vi "rcm_pose.vi"(6 "Adjust RCM":bool=TRUE, 9 "Goal positions":sgl[][](array[numeric]), 11 "Nominal positions":sgl[][](array[numeric])) -> (2 "Goal pose (handle basis)":T1 format="%#_4g")   [LabVIEW 2013]
uses:
  <vilib>/Analysis/Matrix/Datatypes/RealMatrix.ctl
  <vilib>/Analysis/baseanly.llb/A x Vector.vi
  utilities/labview/norm_vec_single.vi
  <vilib>/Analysis/baseanly.llb/Real Dot Product.vi
  <vilib>/Analysis/baseanly.llb/Real A x B.vi
  <vilib>/Analysis/NI_AALBase.lvlib
  <vilib>/Analysis/Matrix/NI_Matrix.lvlib
panel:
  out "Adjusted RCM Goal":sgl[](array[numeric])
  out "Calibrated length":sgl
  out "Goal length":sgl
  out "Adjustment unit vector":dbl[](array[numeric]) format="%.2f"
  out "RCM transform":T1 format="%#_3f"
  out "Relative motion (RCM)":T1 format="%#_3f"
  out "Goal in RCM coords":sgl[][](array[numeric])
  # "Debugging:"
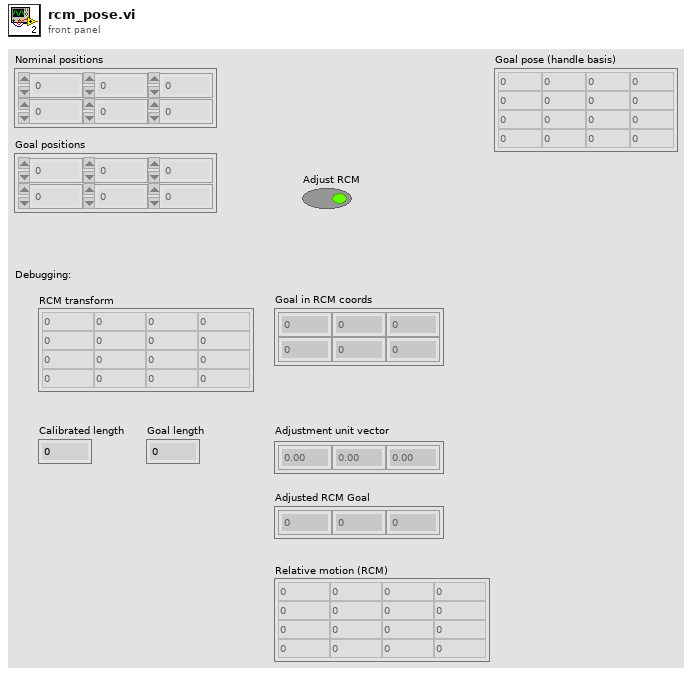
[diagram p1: front panel]
types:
  T1 = typedef "NI_Matrix.lvlib/RealMatrix.ctl" = dbl[][]
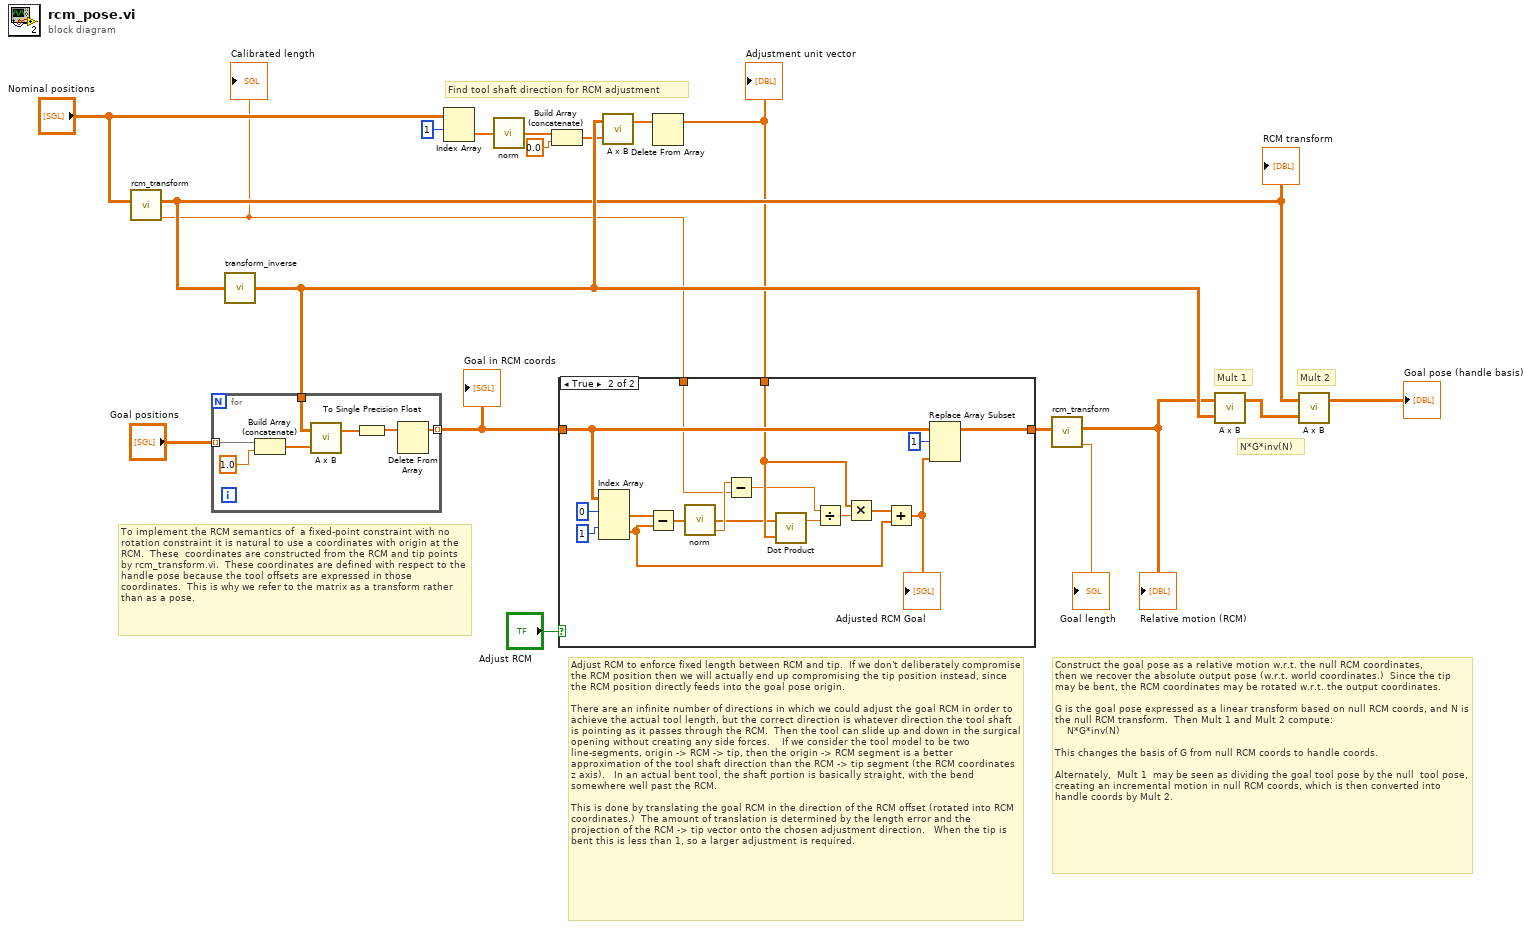
[diagram p0: block diagram]
diagram:
  # "To implement the RCM semantics of  a fixed-point constraint with no rotation constraint it is natural to use a coordinates with origin at the RCM.  These  coordinates are constructed from the RCM and tip points by rcm_transform.vi.  These coordinates are defined with respect to the handle pose because the tool offsets are expressed in those coordinates.  This is why we refer to the matrix as a transform rather than as a pose."
  # "N*G*inv(N)"
  # "Mult 2"
  # "Mult 1"
  # "Find tool shaft direction for RCM adjustment"
  # "Adjust RCM to enforce fixed length between RCM and tip.  If we don't deliberately compromise the RCM position then we will actually end up compromising the tip position instead, since the RCM position directly feeds into the goal pose origin.\n\nThere are an infinite number of directions in which we could adjust the goal RCM in order to achieve the actual tool length, but the correct direction is whatever direction the tool shaft  is pointing as it passes through the RCM.  Then the tool can slide up and down in the surgical opening without creating any side forces.    If we consider the tool model to be two line-segments, origin -> RCM -> tip, then the origin -> RCM segment is a better approximation of the tool shaft direction than the RCM -> tip segment (the RCM coordinates z axis).   In an actual bent tool, the shaft portion is basically straight, with the bend somewhere well past the RCM. \n\nThis is done by translating the goal RCM in the direction of the RCM offset (rotated into RCM coordinates.)  The amount of translation is determined by the length error and the projection of the RCM -> tip vector onto the chosen adjustment direction.   When the tip is bent this is less than 1, so a larger adjustment is required."
  # "Construct the goal pose as a relative motion w.r.t. the null RCM coordinates, \nthen we recover the absolute output pose (w.r.t. world coordinates.)  Since the tip may be bent, the RCM coordinates may be rotated w.r.t. the output coordinates. \n\nG is the goal pose expressed as a linear transform based on null RCM coords, and N is the null RCM transform.  Then Mult 1 and Mult 2 compute:\n    N*G*inv(N)\n \nThis changes the basis of G from null RCM coords to handle coords.  \n\nAlternately,  Mult 1  may be seen as dividing the goal tool pose by the null  tool pose, creating an incremental motion in null RCM coords, which is then converted into handle coords by Mult 2."
  n1 = call "rcm_transform.vi"("Tip and RCM"="Nominal positions") -> ("Length"=w8:sgl, "RCM transform"=w15:T1)  [unwired: 9 in]
  "RCM transform" <- w15
  "Calibrated length" <- w8
  n2 = call "transform_inverse.vi"("Transform"=w15) -> ("Inverse transform"=w18:T1)
  n3 = for {
    tunnel: [w26] -> w17 mode=indexing
    tunnel: "Goal positions" -> [w23] mode=indexing
    tunnel: w18 -> [w22]
    n4 = Build Array (concatenate)(w23, sgl 1.0) -> (w20:sgl[])
    n5 = call-poly <vilib>:"A x B.vi"("Vector"=w20, "A"=w22) -> ("A x Vector"=w21:dbl[])  [unwired: 1 out]
    n6 = To Single Precision Float(number=w21) -> (single precision float=w25:sgl[])
    n7 = Delete From Array(array=w25) -> (array with subset deleted=w26:sgl[])  [unwired: 2 in, 1 out]
  }
  "Goal in RCM coords" <- w17
  n8 = Index Array(array="Nominal positions", index (row)=1) -> (element=w10:sgl[])  [unwired: 1 in]
  n9 = call-poly "norm.vi"("vector"=w10) -> ("normalized vector"=w11:sgl[])  [unwired: 3 in, 1 out]
  n10 = Build Array (concatenate)(w11, sgl 0.0 ("magnitude")) -> (w13:sgl[])
  n11 = call-poly <vilib>:"A x B.vi"("Vector"=w13, "A"=w18) -> ("A x Vector"=w6:dbl[])  [unwired: 1 out]
  n12 = Delete From Array(array=w6) -> (array with subset deleted=w7:dbl[])  [unwired: 2 in, 1 out]
  "Adjustment unit vector" <- w7
  n13 = case shown="True" "Adjust RCM" {
    tunnel: w17 -> [w27 w44]
    tunnel: w8 -> [_ w41]
    tunnel: w7 -> [_ w40]
    tunnel: [w27 w39] -> w5
    frame False {
    }
    frame True {
      n14 = Index Array(array=w44, index (row) #1=0 ("index (row)"), index (row) #2=1 ("index (row)")) -> (element #1=w30:sgl[], element #2=w37:sgl[])  [unwired: 2 in]
      n15 = Subtract(x=w30, y=w37) -> (x-y=w31:sgl[])
      n16 = call-poly "norm.vi"("vector"=w31) -> ("magnitude"=w42:sgl, "normalized vector"=w32:sgl[])  [unwired: 3 in]
      n17 = Subtract(x=w42, y=w41) -> (x-y=w33:sgl)
      n18 = call-poly <vilib>:"Dot Product.vi"("Y Vector"=w40, "X Vector"=w32) -> ("X * Y"=w34:dbl)  [unwired: 1 out]
      n19 = Divide(x=w33, y=w34) -> (x/y=w35:dbl)
      n20 = Multiply ("Multiply.vi")(x=w40, y=w35) -> (x*y=w36:dbl[])
      n21 = Add(x=w36, y=w37) -> (x+y=w43:dbl[])
      "Adjusted RCM Goal" <- w43
      n22 = Replace Array Subset(array=w44, new element=w43, index (row)=1) -> (w39:sgl[][])  [unwired: 1 in]
    }
  }
  n23 = call "rcm_transform.vi"("Tip and RCM"=w5) -> ("Length"=→"Goal length":sgl, "RCM transform"=w2:T1)  [unwired: 9 in]
  "Relative motion (RCM)" <- w2
  n24 = call-poly <vilib>:"A x B.vi"("B"=w18, "A"=w2) -> ("A x B"=w3:T1)  [unwired: 1 out]
  n25 = call-poly <vilib>:"A x B.vi"("B"=w3, "A"=w15) -> ("A x B"=→"Goal pose (handle basis)":T1)  [unwired: 1 out]
